vi "Modbus Control.vi"(7 "Modbus Watchdog In":T1, 8 "Error In":errorcluster, 9 "Modbus Holding Registers In":T3={"System Available Capacity (40000)"=600, "System Reserve Percentage (40001)"=200, "System Active Load (40002)"=0, "System Reactive Load (40003)"=0, "Manual Power (40004)"=0, "Manual Current (40005)"=0, "System Watchdog (40006)"=0, "Spot Gen Op Percentage (40007)"=500, "Control Word (40051)"=128, "Clear Faults (40052)"=0} {"Clear Faults (40052)" format="%016b"; "Control Word (40051)" format="%016b"}) -> (0 "Error Out":errorcluster, 2 "Connected?":bool, 5 "Modbus Watchdog Out":T1)   [LabVIEW 2014]
uses:
  eng/trunk/ni/cRIO Master Files/Controls/ModbusHoldingRegisters.ctl
  <userlib>/cRIO Master Files/Controls/ModbusWatchdog.ctl
  <userlib>/cRIO Master Files/Controls/TimerData.ctl
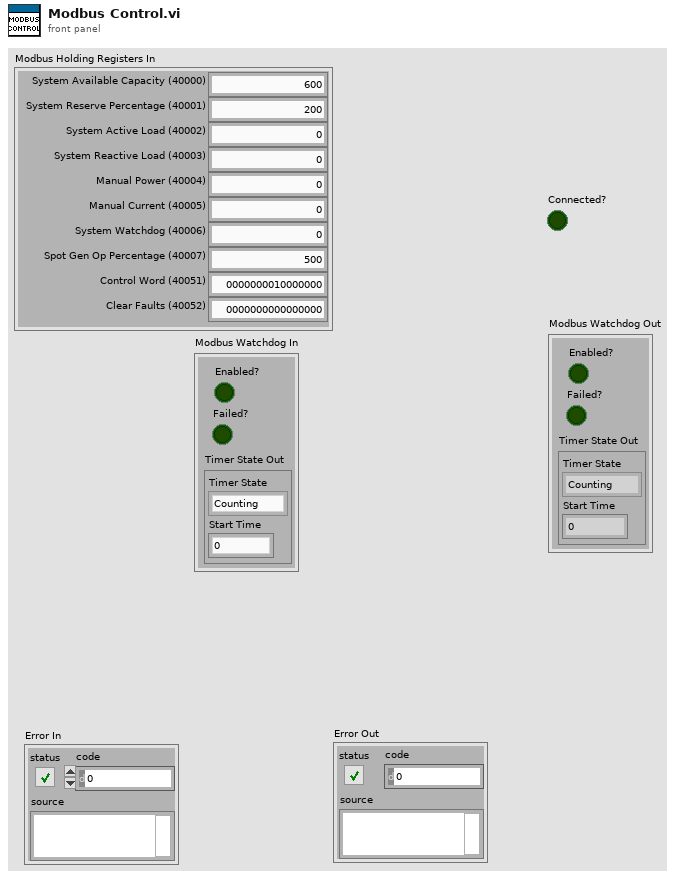
[diagram p1: front panel]
types:
  T1 = typedef "ModbusWatchdog.ctl" = cluster{"Enabled?":bool, "Failed?":bool, "Timer State Out":T2}
  T2 = typedef "TimerData.ctl" = cluster{"Start Time":u32, "Timer State":enum16{"Counting", "Start Timer"}}
  T3 = typedef "ModbusHoldingRegisters.ctl" = cluster{"System Available Capacity (40000)":u16, "System Reserve Percentage (40001)":u16, "System Active Load (40002)":i16, "System Reactive Load (40003)":i16, "Manual Power (40004)":i16, "Manual Current (40005)":i16, "System Watchdog (40006)":u16, "Spot Gen Op Percentage (40007)":u16, "Control Word (40051)":u16, "Clear Faults (40052)":u16}
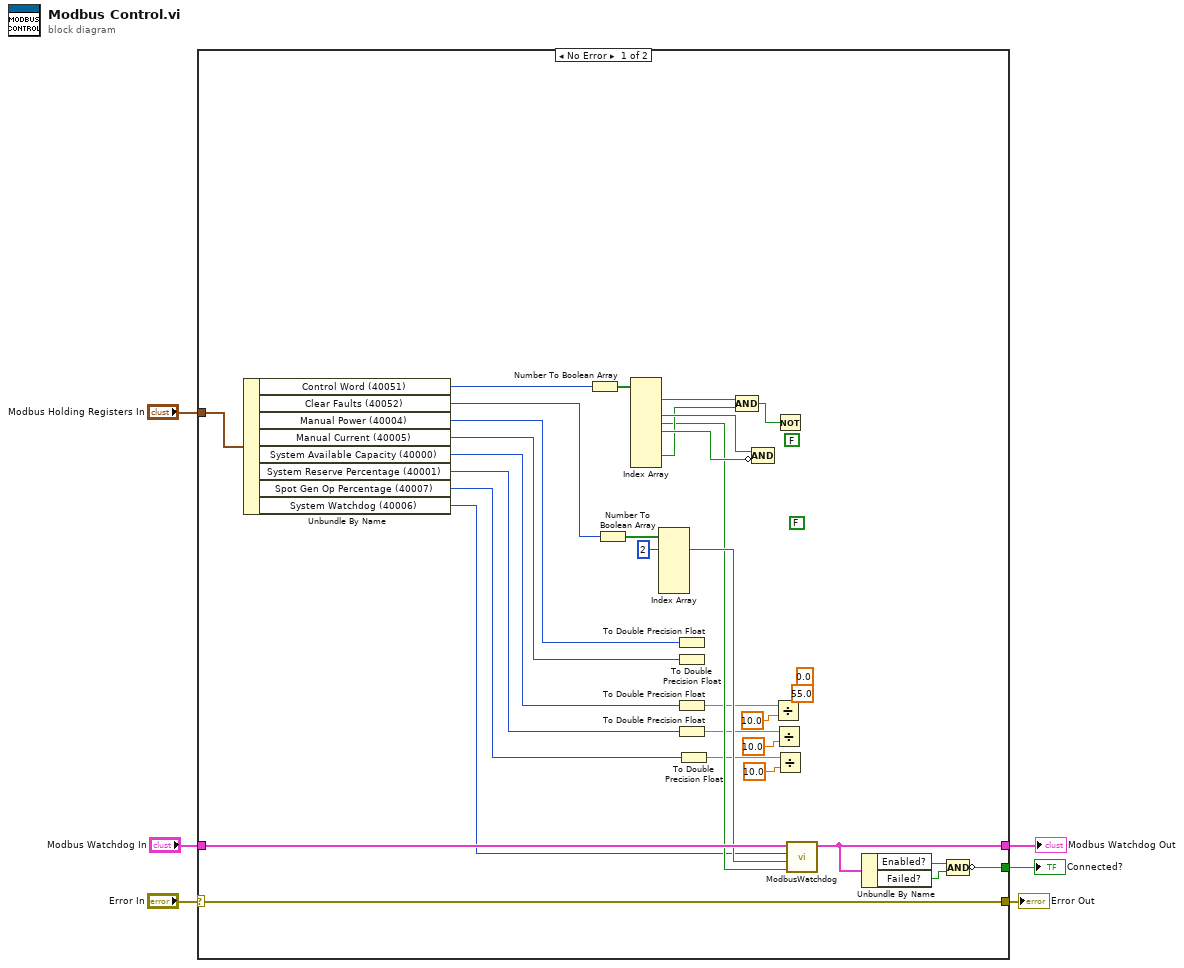
[diagram p0: block diagram]
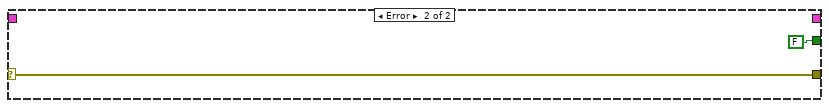
[diagram p2: hidden frame]
diagram:
  n1 = case shown="No Error" "Error In" {
    selector: "Error In" -> [w34 w39]
    tunnel: [w34 w39] -> w5
    tunnel: "Modbus Holding Registers In" -> [w37 _]
    tunnel: "Modbus Watchdog In" -> [w23 _]
    tunnel: [w21 _] -> w2
    tunnel: [w18 FALSE] -> w1
    frame No Error {
      (unwired) 55.0 ("HV Setpoint")
      (unwired) 0.0 ("Charge Control Value")
      (unwired) FALSE ("Charge Control")
      (unwired) FALSE ("Virtual Inertia")
      n2 = Unbundle By Name(w37) -> ("Control Word (40051)"=w36:u16, "Clear Faults (40052)"=w32:u16, "Manual Power (40004)"=w31:i16, "Manual Current (40005)"=w30:i16, "System Available Capacity (40000)"=w16:u16, "System Reserve Percentage (40001)"=w12:u16, "Spot Gen Op Percentage (40007)"=w7:u16, "System Watchdog (40006)"=w10:u16)
      n3 = Number To Boolean Array(number=w36) -> (Boolean array=w35:bool[])
      n4 = Number To Boolean Array(number=w32) -> (Boolean array=w29:bool[])
      n5 = Index Array(array=w35) -> (element #1=w24:bool, element #3=w27:bool, element #4=w17:bool, element #5=w26:bool, element #8=w25:bool)  [unwired: 9 in, 4 out]
      n6 = Index Array(array=w29, index #1=2 ("index")) -> (element #1=w22:bool)  [unwired: 5 in, 5 out]
      n7 = To Double Precision Float(number=w31) -> ()  [unwired: 1 out]
      n8 = To Double Precision Float(number=w30) -> ()  [unwired: 1 out]
      n9 = To Double Precision Float(number=w16) -> (double precision float=w15:dbl)
      n10 = To Double Precision Float(number=w12) -> (double precision float=w11:dbl)
      n11 = To Double Precision Float(number=w7) -> (double precision float=w8:dbl)
      n12 = Compound Arithmetic op=AND(w24, w25) -> (w33:bool)
      n13 = Compound Arithmetic op=AND(w27, invert w26) -> ()  [unwired: 1 out]
      n14 = Divide(x=w15, y=10.0) -> ()  [unwired: 1 out]
      n15 = Divide(x=w11, y=10.0) -> ()  [unwired: 1 out]
      n16 = Not(x=w33) -> ()  [unwired: 1 out]
      n17 = Divide(x=w8, y=10.0) -> ()  [unwired: 1 out]
      n18 = call "ModbusWatchdog.vi"("Enable Watchdog?"=w17, "Reset Watchdog?"=w22, "System Watchdog (40006)"=w10, "Modbus Watchdog In"=w23) -> ("Modbus Watchdog Out"=w21:T1)  [unwired: 7 in]
      n19 = Unbundle By Name(w21) -> ("Enabled?"=w20:bool, "Failed?"=w19:bool)
      n20 = Compound Arithmetic op=AND(w20, w19) -> (invert w18:bool)
    }
    frame Error {
    }
  }
  "Error Out" <- w5
  "Modbus Watchdog Out" <- w2
  "Connected?" <- w1
